vi "GlobalLB.vi"() -> ()   [LabVIEW 2012]
panel:
  out "LB status":bool[](array[boolean])=[TRUE, TRUE]
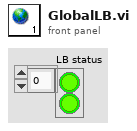
[diagram p1: front panel]
diagram:
